vi "Self-Test.vi"(8 "error in (no error)":errorcluster, 11 "SMO.Instrument":refnum<class "SMO.InstrumentDriver.lvclass">) -> (0 "error out":errorcluster, 3 "SMO.Instrument out":refnum<class "SMO.InstrumentDriver.lvclass">)   [LabVIEW 2013, in "SMO.InstrumentDriver.lvclass"]
doc: "---------------------------------------------------------------\nJKI State Machine Objects™\nhttp://jki.net/state-machine-objects/\nCopyright (C) 2005-2015, JKI <info@jki.net>\nALL RIGHTS RESERVEDJKI State Machine Objects (SMO) 1.0.0.5\nJKI - JKI\nCopyright (c) 2016, JKI"
uses:
  SMO.InstrumentDriver.lvclass
panel:
  # "For instructions on how to use the JKI State Machine Objects, examples and video tutorials, visit:\nhttp://jki.net/state-machine-objects/\n\nJKI State Machine Objects™\nhttp://jki.net/state-machine-objects/\nCopyright (C) 2005-2015, JKI <info@jki.net>\nALL RIGHTS RESERVED"
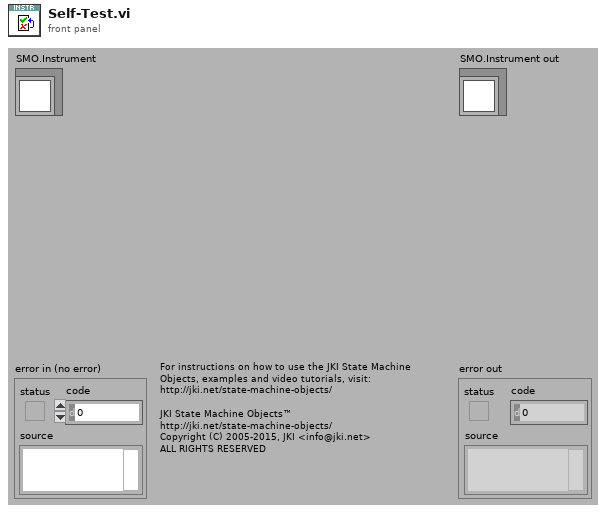
[diagram p1: front panel]
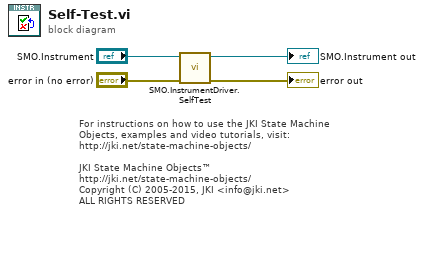
[diagram p0: block diagram]
diagram:
  # "For instructions on how to use the JKI State Machine Objects, examples and video tutorials, visit:\nhttp://jki.net/state-machine-objects/\n\nJKI State Machine Objects™\nhttp://jki.net/state-machine-objects/\nCopyright (C) 2005-2015, JKI <info@jki.net>\nALL RIGHTS RESERVED"
  n1 = call-dynamic "SMO.InstrumentDriver.SelfTest.vi"("error in (no error)"="error in (no error)", "SMO.Instrument"="SMO.Instrument") -> ("error out"=→"error out":errorcluster, "SMO.Instrument out"=→"SMO.Instrument out":refnum<class "SMO.InstrumentDriver.lvclass">)  [unwired: 8 in]
